vi "Configure Input Settings.vi"(0 "VISA resource name":refnum<visa-resource-name>, 1 "Filter (F: Off)":bool, 2 "Filter Points (8)":dbl=8.0, 3 "Filter Window (1 %)":dbl=1.0, 5 "Input (0:A)":u16(ring) items=["A", "B"], 7 "Sensor Type (0:Silicon Diode)":u16(ring) items=["Silicon Diode", "GaAlAs Diode", "100 Ohm Platinum/250", "100 Ohm Platinum/500", "1000 Ohm Platinum", "NTC RTD", "Thermocouple 25 mV", "Thermocouple 50 mV", "2.5 V, 1 mA", "7.5 V, 1 mA"], 9 "Curve (0:None)":u16(ring) items=["None"=0, "DT-470"=1, "DT-670"=2, "DT-500-D"=3, "DT-500-E1"=4, "PT-100"=6, "PT-1000"=7, "RX-102A-AA"=8, "RX-202A-AA"=9, "Type K"=12, "Type E"=13, "Type T"=14, "AuFe 0.03%"=15, "AuFe 0.07%"=16, "User 21"=21, "User 22"=22, "User 23"=23, "User 24"=24, "User 25"=25, "User 26"=26, "User 27"=27, "User 28"=28, "User 29"=29, "User 30"=30, "User 31"=31], 11 "error in (no error)":errorcluster, 12 "Compensation (F: Off)":bool) -> (4 "VISA resource name out":refnum<visa-resource-name>, 15 "error out":errorcluster)   [LabVIEW 2019, in "Lake Shore 325.lvlib"]
doc: "This VI configures the sensor input settings and input filter. The Model 325 supports a variety of temperature sensors sold by Lake Shore and other manufacturers. An appropriate sensor type must be selected for each of the two inputs. If the exact sensor model is not shown, use the sensor input performance chart in section 4 of the 325 User's Manual."
uses:
  Lake Shore 325.lvlib
  Instance           1 32Saved   Configure Input Settings .vi
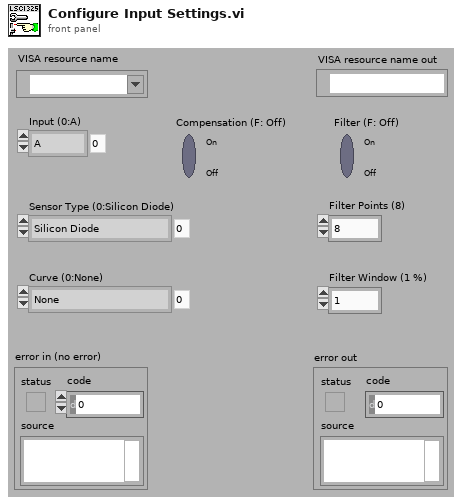
[diagram p1: front panel]
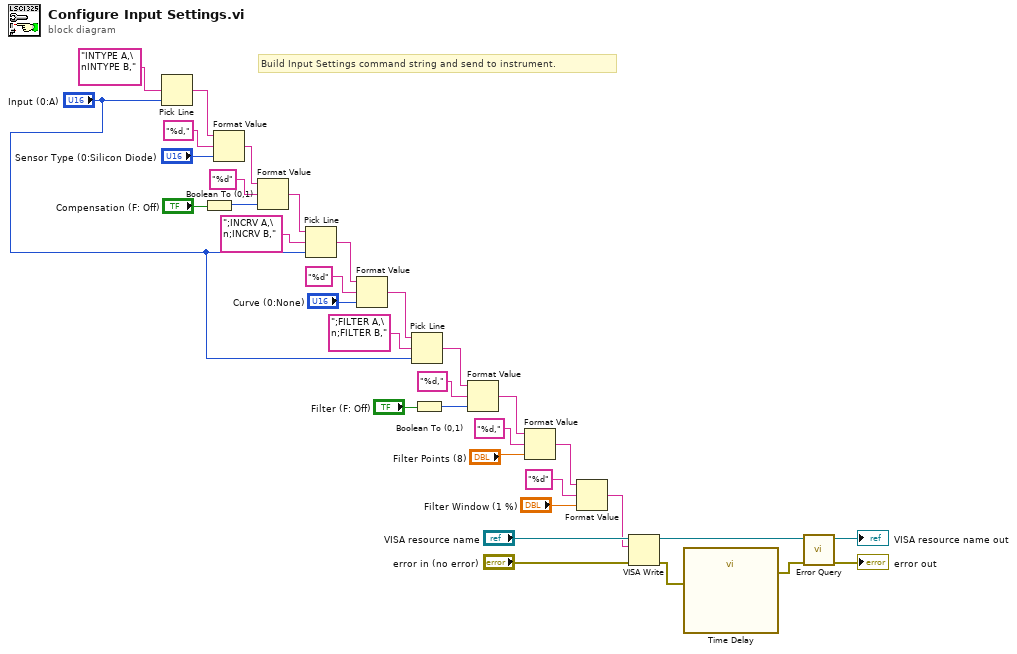
[diagram p0: block diagram]
diagram:
  # "Build Input Settings command string and send to instrument."
  n1 = Pick Line(multi-line string="INTYPE A,\nINTYPE B,", line index="Input (0:A)") -> (output string=w24:string)  [unwired: 1 in]
  n2 = Boolean To (0,1)(Boolean="Compensation (F: Off)") -> (0, 1=w20:i16)
  n3 = Format Value(string ("")=w24, format string="%d,", value (0)="Sensor Type (0:Silicon Diode)") -> (output string=w21:string)
  n4 = Format Value(string ("")=w21, format string="%d", value (0)=w20) -> (output string=w19:string)
  n5 = Pick Line(string ("")=w19, multi-line string=";INCRV A,\n;INCRV B,", line index="Input (0:A)") -> (output string=w17:string)
  n6 = Format Value(string ("")=w17, format string="%d", value (0)="Curve (0:None)") -> (output string=w16:string)
  n7 = Pick Line(string ("")=w16, multi-line string=";FILTER A,\n;FILTER B,", line index="Input (0:A)") -> (output string=w11:string)
  n8 = Boolean To (0,1)(Boolean="Filter (F: Off)") -> (0, 1=w12:i16)
  n9 = Format Value(string ("")=w11, format string="%d,", value (0)=w12) -> (output string=w8:string)
  n10 = Format Value(string ("")=w8, format string="%d,", value (0)="Filter Points (8)") -> (output string=w7:string)
  n11 = Format Value(string ("")=w7, format string="%d", value (0)="Filter Window (1 %)") -> (output string=w4:string)
  n12 = VISA Write(VISA resource name="VISA resource name", write buffer=w4, error in (no error)="error in (no error)") -> (VISA resource name out=w31:refnum<visa-resource-name>, error out=w2:errorcluster)  [unwired: 1 out]
  n13 = call "Time Delay"("error in (no error)"=w2) -> ("error out"=w1:errorcluster)  [unwired: 10 in]
  n14 = call "Error Query.vi"("error in (no error)"=w1, "VISA resource name"=w31) -> ("error out"=→"error out":errorcluster, "VISA resource name out"=→"VISA resource name out":refnum<visa-resource-name>)  [unwired: 7 in, 1 out]
